vi "Variable Servo Fan.vi"() -> ()   [LabVIEW 2009]
uses:
  <vilib>/DAQmx/create/channels.llb/DAQmx Create Channel (AO-Voltage-Basic).vi
  <vilib>/DAQmx/write.llb/DAQmx Write (Analog DBL 1Chan 1Samp).vi
panel:
  in  "stop":bool
  in  "physical channels":tag
  in  "Speed":dbl(slide) scale=0.0..5.0
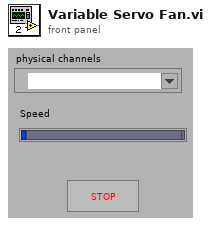
[diagram p1: front panel]
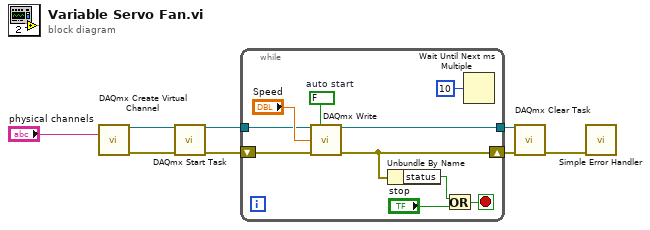
[diagram p0: block diagram]
diagram:
  n1 = call-poly <vilib>:"DAQmx Create Virtual Channel.vi"("physical channels"="physical channels") -> ("task out"=w7:refnum<k21>, "error out"=w6:errorcluster)  [unwired: 13 in]
  n2 = call <vilib>:"DAQmx Start Task.vi"("task/channels in"=w7, "error in"=w6) -> ("task out"=w5:refnum<k21>, "error out"=w4:errorcluster)  [unwired: 12 in]
  n3 = while {
    tunnel: w5 -> [w16]
    tunnel: [w14] -> w3
    shift-right: [w12] -> w1
    shift-left: w4 -> [w15]
    stop <- w9 stop-if-true
    w17 = FALSE  # auto start
    n4 = call-poly <vilib>:"DAQmx Write.vi"("task/channels in"=w16, "auto start"=w17, "data"="Speed", "error in"=w15) -> ("task out"=w14:refnum<k21>, "error out"=w12:errorcluster)  [unwired: 9 in, 1 out]
    n5 = Unbundle By Name "Unbundle By Name"(w12) -> ("status"=w11:bool)
    n6 = Or(x=w11, y="stop") -> (x .or. y?=w9:bool)
    n7 = Wait Until Next ms Multiple(millisecond multiple=u32 10) -> ()  [unwired: 1 out]
  }
  n8 = call <vilib>:"DAQmx Clear Task.vi"("task in"=w3, "error in"=w1) -> ("error out"=w2:errorcluster)  [unwired: 13 in]
  n9 = call <vilib>:"Simple Error Handler.vi"("error in (no error)"=w2) -> ()  [unwired: 4 in, 5 out]
